vi "linear fit left.vi"(6 "# of samples":dbl, 11 "Left in":i8) -> (3 "Left out":i8)   [LabVIEW 2012, in "BlockParty4150.lvrbt"]
uses:
  BlockParty4150.lvrbt
  <vilib>/NXT/Dual Mode Library/prims/inRangeAndCoerce/inRangeAndCoerce_int.vi
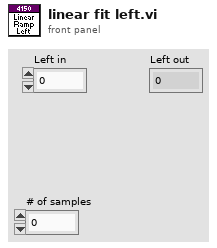
[diagram p1: front panel]
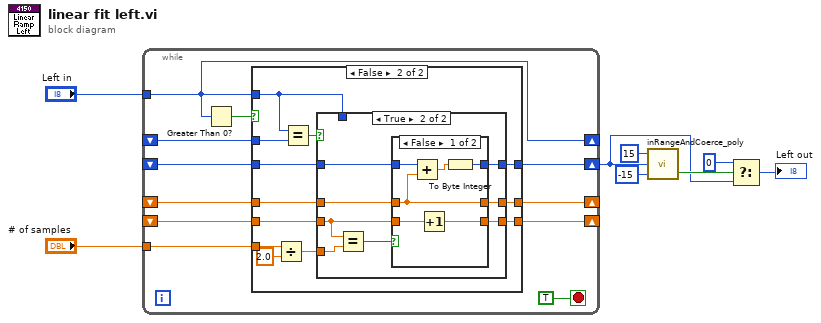
[diagram p0: block diagram]
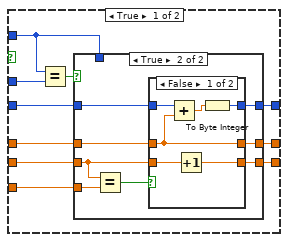
[diagram p2: hidden frame]
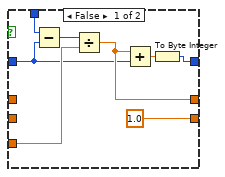
[diagram p3: hidden frame]
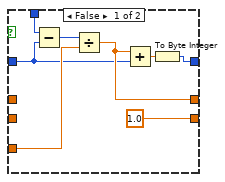
[diagram p5: hidden frame]
diagram:
  n1 = while {
    tunnel: "Left in" -> [w10]
    shift-right: [w10] -> _
    shift-left: _ -> [w19]
    shift-right: [w16] -> w3
    shift-left: _ -> [w18]
    shift-right: [w14] -> _
    shift-left: _ -> [w15]
    shift-right: [w13] -> _
    shift-left: _ -> [w12]
    tunnel: "# of samples" -> [w17]
    stop <- TRUE stop-if-true
    n2 = Greater Than 0?(x=w10) -> (x > 0?=w9:bool)
    n3 = case shown="False" w9 {
      tunnel: w19 -> [w29 w66]
      tunnel: w10 -> [w27 w64]
      tunnel: w18 -> [w26 w63]
      tunnel: w17 -> [w25 w57]
      tunnel: [w24 w62] -> w16
      tunnel: w15 -> [w23 w61]
      tunnel: [w22 w60] -> w14
      tunnel: [w21 w59] -> w13
      tunnel: w12 -> [w20 w58]
      frame True {
        n4 = Equal?(x=w27, y=w29) -> (x = y?=w28:bool)
        n5 = case shown="True" w28 {
          tunnel: w27 -> [w37 _]
          tunnel: w26 -> [w30 w45]
          tunnel: w25 -> [w35 w41]
          tunnel: [w33 w44] -> w24
          tunnel: w23 -> [_ w43]
          tunnel: [w32 w42] -> w22
          tunnel: [1.0 w38] -> w21
          tunnel: w20 -> [_ w39]
          frame False {
            n6 = Subtract(x=w37, y=w30) -> (x-y=w36:i8)
            n7 = Divide(x=w36, y=w35) -> (x/y=w32:dbl)
            n8 = Add(x=w32, y=w30) -> (x+y=w34:dbl)
            n9 = To Byte Integer(number=w34) -> (8bit integer=w33:i8)
          }
          frame True {
            n10 = Equal?(x=w39, y=w41) -> (x = y?=w40:bool)
            n11 = case shown="False" w40 {
              tunnel: w45 -> [w51 w52]
              tunnel: [w49 w52] -> w44
              tunnel: w43 -> [w48 w54]
              tunnel: [w48 w54] -> w42
              tunnel: w39 -> [w47 w53]
              tunnel: [w46 w53] -> w38
              frame False {
                n12 = Add(x=w51, y=w48) -> (x+y=w50:dbl)
                n13 = Increment(x=w47) -> (x+1=w46:dbl)
                n14 = To Byte Integer(number=w50) -> (8bit integer=w49:i8)
              }
              frame True {
              }
            }
          }
        }
      }
      frame False {
        n15 = Divide(x=w57, y=2.0) -> (x/y=w56:dbl)
        n16 = Equal?(x=w64, y=w66) -> (x = y?=w65:bool)
        n17 = case shown="True" w65 {
          tunnel: w64 -> [w74 _]
          tunnel: w63 -> [w67 w82]
          tunnel: w56 -> [w72 w78]
          tunnel: [w70 w81] -> w62
          tunnel: w61 -> [_ w80]
          tunnel: [w69 w79] -> w60
          tunnel: [1.0 w75] -> w59
          tunnel: w58 -> [_ w76]
          frame False {
            n18 = Subtract(x=w74, y=w67) -> (x-y=w73:i8)
            n19 = Divide(x=w73, y=w72) -> (x/y=w69:dbl)
            n20 = Add(x=w69, y=w67) -> (x+y=w71:dbl)
            n21 = To Byte Integer(number=w71) -> (8bit integer=w70:i8)
          }
          frame True {
            n22 = Equal?(x=w76, y=w78) -> (x = y?=w77:bool)
            n23 = case shown="False" w77 {
              tunnel: w82 -> [w88 w89]
              tunnel: [w86 w89] -> w81
              tunnel: w80 -> [w85 w91]
              tunnel: [w85 w91] -> w79
              tunnel: w76 -> [w84 w90]
              tunnel: [w83 w90] -> w75
              frame False {
                n24 = Add(x=w88, y=w85) -> (x+y=w87:dbl)
                n25 = Increment(x=w84) -> (x+1=w83:dbl)
                n26 = To Byte Integer(number=w87) -> (8bit integer=w86:i8)
              }
              frame True {
              }
            }
          }
        }
      }
    }
  }
  n27 = call-poly <vilib>:"inRangeAndCoerce_poly.vi"("lower limit"=-15, "x"=w3, "upper limit"=15) -> ("In Range?"=w4:bool)  [unwired: 1 out]
  n28 = Select(t=i8 0, s=w4, f=w3) -> (s? t:f=→"Left out":i8)
